vi "set_Event.vi"(8 "error in (no error)":errorcluster, 10 "HGF_Event":refnum<class "HGF_Event.lvclass">, 11 "HGF_PVObjectPublisher":refnum<class "HGF_PVObjectPublisher.lvclass">) -> (0 "error out":errorcluster, 3 "dup HGF_PVObjectPublisher":refnum<class "HGF_PVObjectPublisher.lvclass">)   [LabVIEW 2014, in "HGF_BaseClasses.lvlib" / "HGF_PVObjectPublisher.lvclass"]
doc: "Set HGF_Event object."
uses:
  HGF_PVObjectPublisher.lvclass
  HGF_Event/HGF_Event.lvclass
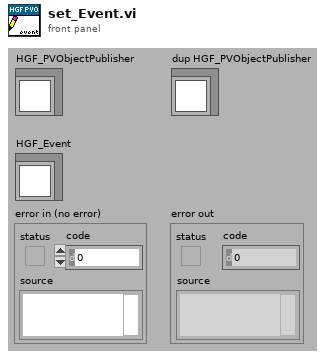
[diagram p1: front panel]
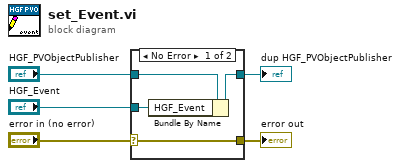
[diagram p0: block diagram]
diagram:
  n1 = case shown="No Error" "error in (no error)" {
    selector: "error in (no error)" -> [w9 w10]
    tunnel: [w9 w10] -> w4
    tunnel: [w7 w11] -> w2
    tunnel: "HGF_PVObjectPublisher" -> [w8 w11]
    tunnel: "HGF_Event" -> [w6 _]
    frame No Error {
      n2 = Bundle By Name(cluster=w8, "HGF_Event"=w6) -> (w7:refnum<class "HGF_PVObjectPublisher.lvclass">)
    }
    frame Error {
    }
  }
  "error out" <- w4
  "dup HGF_PVObjectPublisher" <- w2
